vi "Config.vi"(8 "error in (no error)":errorcluster, 10 "Setting":variant, 11 "FPGA:R-Series in":refnum<class "R-Series.lvclass">) -> (0 "error out":errorcluster, 3 "FPGA:R-Series out":refnum<class "R-Series.lvclass">)   [LabVIEW 2025, in "FPGA.lvlib" / "R-Series.lvclass"]
uses:
  R-Series.lvclass
  C:/Working copy/tss/Plugin/Engines/FPGA/FPGA Instrument/FPGA Instrument.lvclass
  FPGA configuration/FPGA configuration.lvclass
  C:/Users/Public/Documents/Sandia National Labs/TSS Plugin/Abstract Engine.lvlibp/Plugin/Abstract/Instrument configuration/Instrument configuration.lvclass
  R-Series.lvclass/R-Series.ctl
  FPGA configuration/Read FPGA Setting.vi
  Users/Public/Documents/Sandia National Labs/TSS Plugin/Abstract Engine.lvlibp/Plugin/Abstract/Instrument configuration/Read Instrument Setting.vi
  Users/Public/Documents/Sandia National Labs/TSS Plugin/CEF.lvlibp/serializable configuration/CEF_serializable configuration.lvclass
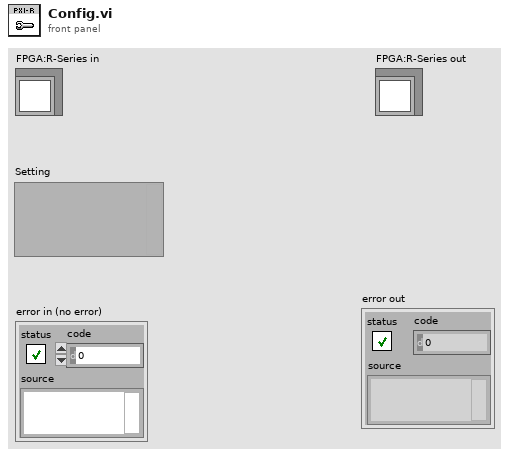
[diagram p1: front panel]
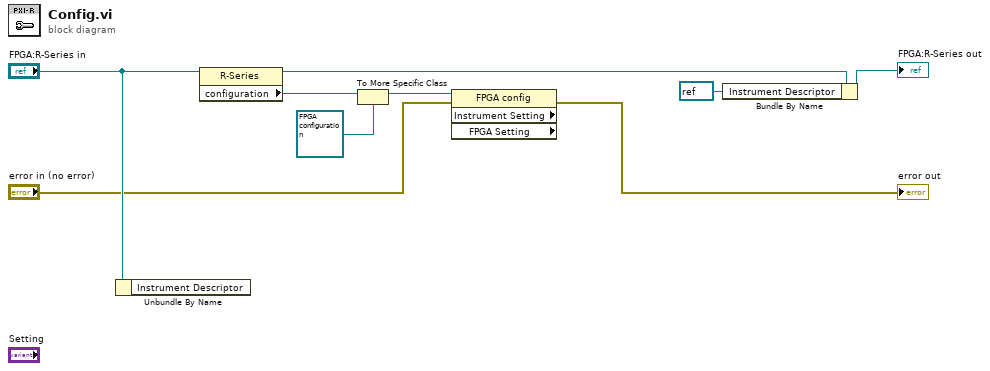
[diagram p0: block diagram]
diagram:
  n1 = Unbundle By Name("FPGA:R-Series in") -> ()  [unwired: 1 out]
  n2 = property class="R-Series"(reference="FPGA:R-Series in") -> (reference out=w6:refnum<class "R-Series.lvclass">, "configuration"=w7:refnum<class "CEF_serializable configuration.lvclass">)  [unwired: 1 in, 1 out]
  n3 = To More Specific Class(target class=refnum<class "FPGA configuration.lvclass"> refnum ("DMM.lvlib:DMM configuration.lvclass"), reference=w7) -> (specific class reference=w8:refnum<class "FPGA configuration.lvclass">)  [unwired: 1 in, 1 out]
  n4 = property class="FPGA config" props=["Instrument Setting", "FPGA Setting"](reference=w8, error in="error in (no error)") -> (error out=→"error out":errorcluster)  [unwired: 3 out]
  n5 = Bundle By Name(cluster=w6, "Instrument Descriptor"=refnum<k15> refnum) -> (→"FPGA:R-Series out":refnum<class "R-Series.lvclass">)
